vi "TurnToDegrees.vi"(8 "error in":errorcluster, 11 "Angle":dbl) -> (0 "error out":errorcluster)   [LabVIEW 2016]
uses:
  Robot Global Data.vi
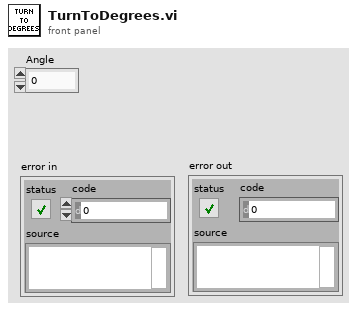
[diagram p1: front panel]
types:
  T1 = cluster{" Proportional Gain":dbl, "Integral Time":dbl, "Derivative Time":dbl}
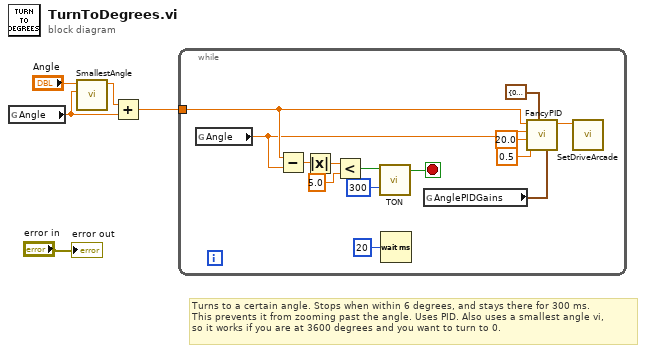
[diagram p0: block diagram]
diagram:
  # "Turns to a certain angle. Stops when within 6 degrees, and stays there for 300 ms. \nThis prevents it from zooming past the angle. Uses PID. Also uses a smallest angle vi,\nso it works if you are at 3600 degrees and you want to turn to 0."
  n1 = global read "Robot Global Data.vi" "Angle"() -> (w2:dbl)
  n2 = call "SmallestAngle.vi"("Angle B"=w2, "Angle A"="Angle") -> ("Smallest B to A"=w3:dbl)  [unwired: 9 in]
  n3 = Add(x=w3, y=w2) -> (x+y=w1:dbl)
  n4 = while {
    tunnel: w1 -> [w14]
    stop <- w7 stop-if-true
    n5 = global read "Robot Global Data.vi" "Angle"() -> (w13:dbl)
    n6 = Subtract(x=w14, y=w13) -> (x-y=w12:dbl)
    n7 = Absolute Value(x=w12) -> (abs(x)=w11:dbl)
    n8 = Less?(x=w11, y=5.0) -> (x < y?=w9:bool)
    n9 = call "TON.vi"("Time Limit"=u32 300, "Input"=w9) -> ("Output"=w7:bool)  [unwired: 9 in]
    n10 = Wait (ms)(milliseconds to wait=u32 20) -> ()  [unwired: 1 out]
    n11 = global read "Robot Global Data.vi" "AnglePIDGains"() -> (w6:T1)
    n12 = call "FancyPID.vi"("Gains"=w6, "Range"=cluster{"output high":dbl, "output low":dbl} {"output high"=0.7, "output low"=-0.7}, "Disable Range"=0.5, "Integral Range"=20.0, "Process variable"=w13, "Setpoint"=w14) -> ("output"=w16:dbl)  [unwired: 5 in]
    n13 = call "SetDriveArcade.vi"("Turn"=w16) -> ()  [unwired: 10 in, 1 out]
  }
  "error out" <- "error in"
